vi "Get_Next_Data.vi"(8 "error in (no error)":errorcluster caption="entrée d'erreur (pas d'erreur)", 11 "Firebase Altyor en entrée":refnum<class "Firebase Altyor.lvclass">) -> (0 "error out":errorcluster caption="sortie d'erreur", 3 "Firebase Altyor en sortie":refnum<class "Firebase Altyor.lvclass">)   [LabVIEW 2020, in "Library Instrument & Equipement.lvlib" / "Library FireBase.lvlib" / "Firebase Altyor.lvclass"]
doc: "Returns data according to Value_To_Find Use Nb_To_Read to determine the number to read\nPlease initialise the following values before use the VI\n - Name BDD\n - Value to find\n - Document\n - API Key"
uses:
  Firebase Altyor.lvclass
  Firebase Altyor.lvclass/Firebase Altyor.ctl
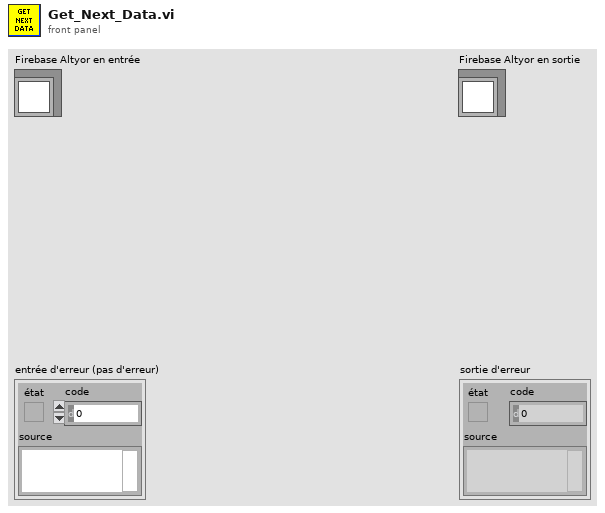
[diagram p1: front panel]
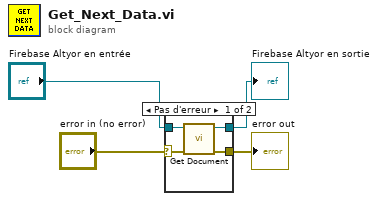
[diagram p0: block diagram]
diagram:
  n1 = case shown="Pas d'erreur" "error in (no error)" {
    selector: "error in (no error)" -> [w8 w10]
    tunnel: [w5 w10] -> w3
    tunnel: [w6 w9] -> w1
    tunnel: "Firebase Altyor en entrée" -> [w7 w9]
    frame No Error {
      n2 = call-dynamic "Get Document.vi"("error in (no error)"=w8, "Firebase (Default) en entrée"=w7) -> ("error out"=w5:errorcluster, "Firebase (Default) en sortie"=w6:refnum<class "Firebase Altyor.lvclass">)  [unwired: 8 in]
    }
    frame Error {
    }
  }
  "error out" <- w3
  "Firebase Altyor en sortie" <- w1
